vi "Configure Modulation (Amplitude).vi"(4 "Modulation Depth (100 %)":i32=100 min=0 max=120, 6 "Modulation Frequency (100 Hz)":dbl=100.0, 7 "Enable Amplitude Modulation (T:Enable)":bool=TRUE, 8 "error in (no error)":errorcluster, 9 "Modulation Waveform (Sine)":T1(ring), 10 "AM Source (Internal)":enum16{"Internal", "External"}(ring), 11 "VISA resource name":refnum<visa-resource-name>) -> (0 "error out":errorcluster, 3 "VISA resource name out":refnum<visa-resource-name>)   [LabVIEW 2017, in "Keithley 3390.lvlib"]
doc: "Configures and enables amplitude modulation (AM). In AM, the amplitude of the carrier is varied by the amplitude of the modulating waveform. \n\n<B>Note:</B> The carrier waveform shape and parameters are set by the Configure Waveform VI."
uses:
  Keithley 3390.lvlib
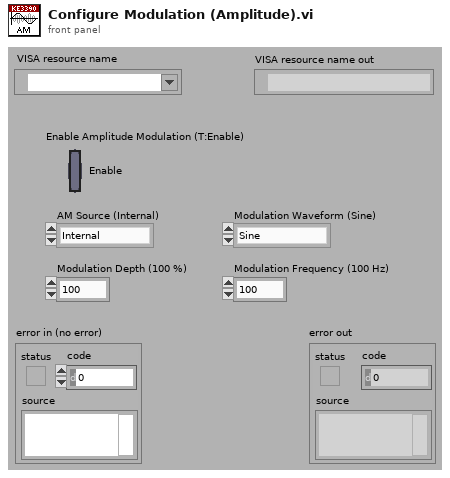
[diagram p1: front panel]
types:
  T1 = enum16{"Sine", "Square", "Ramp", "Negative Ramp", "Triangle", "Noise", "Arbitrary"}
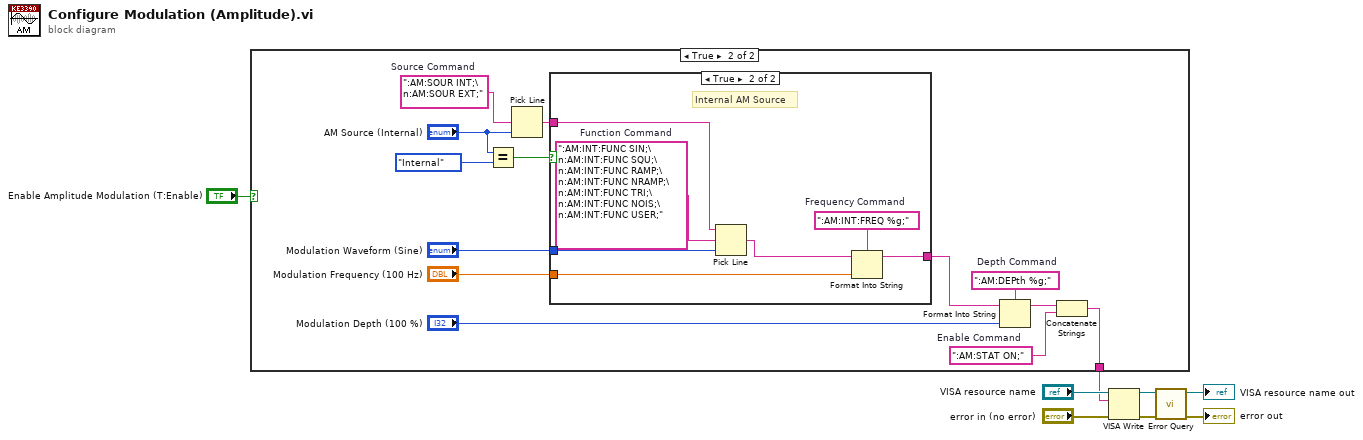
[diagram p0: block diagram]
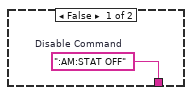
[diagram p2: hidden frame]
diagram:
  n1 = case shown="True" "Enable Amplitude Modulation (T:Enable)" {
    tunnel: [w9 w13] -> w1
    frame False {
      w9 = ":AM:STAT OFF"  # Disable Command
    }
    frame True {
      w12 = ":AM:STAT ON;"  # Enable Command
      w16 = ":AM:DEPth %g;"  # Depth Command
      w18 = ":AM:SOUR INT;\n:AM:SOUR EXT;"  # Source Command
      n2 = Equal?(x="AM Source (Internal)", y=enum16{"Internal", "External"}."Internal") -> (x = y?=w17:bool)
      n3 = Pick Line(multi-line string=w18, line index="AM Source (Internal)") -> (output string=w14:string)  [unwired: 1 in]
      n4 = case shown="True" w17 {
        tunnel: w14 -> [w23 w26]
        tunnel: "Modulation Waveform (Sine)" -> [_ w29]
        tunnel: "Modulation Frequency (100 Hz)" -> [_ w27]
        tunnel: [w23 w24] -> w15
        frame False {
          # "External AM Source"
        }
        frame True {
          w28 = ":AM:INT:FREQ %g;"  # Frequency Command
          w30 = ":AM:INT:FUNC SIN;\n:AM:INT:FUNC SQU;\n:AM:INT:FUNC RAMP;\n:AM:INT:FUNC NRAMP;\n:AM:INT:FUNC TRI;\n:AM:INT:FUNC NOIS;\n:AM:INT:FUNC USER;"  # Function Command
          # "Internal AM Source"
          n5 = Pick Line(string ("")=w26, multi-line string=w30, line index=w29) -> (output string=w25:string)
          n6 = Format Into String(format string=w28, initial string=w25, w27) -> (resulting string=w24:string)  [unwired: 1 in, 1 out]
        }
      }
      n7 = Format Into String(format string=w16, initial string=w15, "Modulation Depth (100 %)") -> (resulting string=w10:string)  [unwired: 1 in, 1 out]
      n8 = Concatenate Strings(w10, w12) -> (w13:string)
    }
  }
  n9 = VISA Write(VISA resource name="VISA resource name", write buffer=w1, error in (no error)="error in (no error)") -> (VISA resource name out=w4:refnum<visa-resource-name>, error out=w3:errorcluster)  [unwired: 1 out]
  n10 = call "Error Query.vi"("error in (no error)"=w3, "VISA resource name"=w4) -> ("error out"=→"error out":errorcluster, "VISA resource name out"=→"VISA resource name out":refnum<visa-resource-name>)  [unwired: 6 in, 2 out]
